vi "Configure Multi DMM.vi"(8 "error in (no error)":errorcluster, 11 "BMC in":refnum<class "BMC.lvclass">) -> (0 "error out":errorcluster, 3 "BMC out":refnum<class "BMC.lvclass">)   [LabVIEW 2012, in "BMC.lvclass"]
uses:
  BMC.lvclass
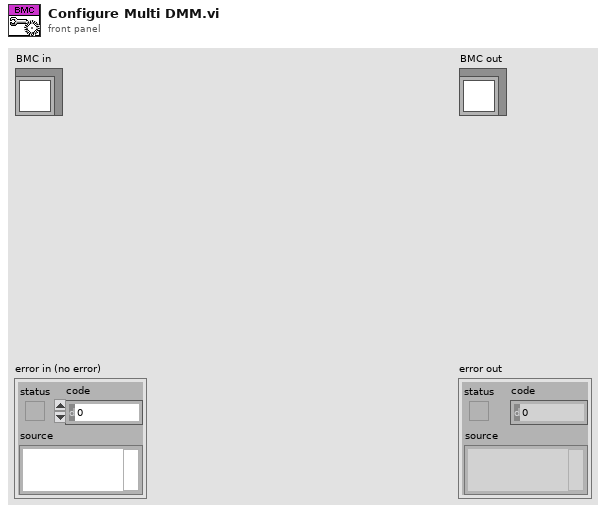
[diagram p1: front panel]
types:
  T1 = enum16{"CIUsb_CONTROL_ASSERT_FRAME_SYNC", "CIUsb_CONTROL_DEASSERT_FRAME_SYNC", "CIUsb_CONTROL_ASSERT_FRESET", "CIUsb_CONTROL_DEASSERT_FRESET", "CIUsb_CONTROL_ASSERT_HV_ENAB", "CIUsb_CONTROL_DEASSERT_HV_ENAB", "CIUsb_CONTROL_ASSERT_LV_SHDN", "CIUsb_CONTROL_DEASSERT_LV_SHDN", "CIUsb_CONTROL_ASSERT_EXT_I2C", "CIUsb_CONTROL_DEASSERT_EXT_I2C", "CIUsb_CONTROL_MINI_MODE"}
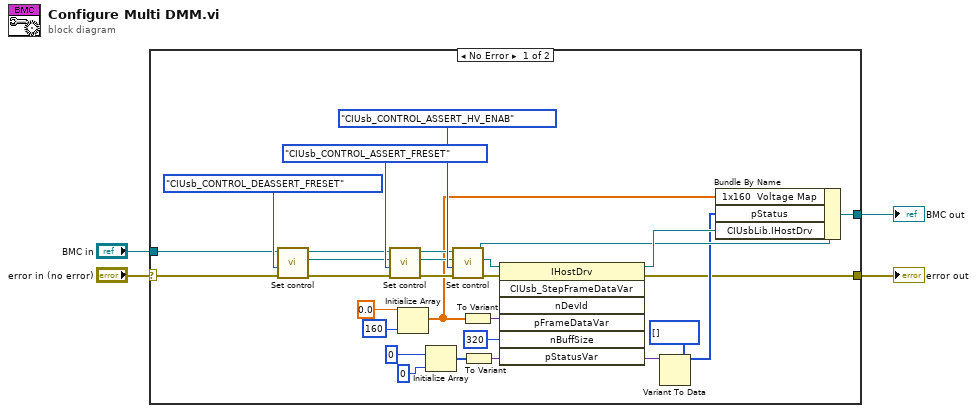
[diagram p0: block diagram]
diagram:
  n1 = case shown="No Error" "error in (no error)" {
    selector: "error in (no error)" -> [w13 w35]
    tunnel: [w12 w35] -> w3
    tunnel: [w10 w34] -> w1
    tunnel: "BMC in" -> [w11 w34]
    frame No Error {
      n2 = call-dynamic "Set control.vi"("BMC in"=w11, "CIUSBLib_SetControl"=T1."CIUsb_CONTROL_DEASSERT_FRESET", "error in (no error)"=w13) -> ("BMC out"=w22:refnum<class "BMC.lvclass">, "CiUsbLib.IHostDrv"=w15:refnum<k7>, "error out"=w26:errorcluster)  [unwired: 5 in]
      n3 = call-dynamic "Set control.vi"("BMC in"=w22, "CIUsbLib.IHostDrv"=w15, "CIUSBLib_SetControl"=T1."CIUsb_CONTROL_ASSERT_FRESET", "error in (no error)"=w26) -> ("BMC out"=w21:refnum<class "BMC.lvclass">, "CiUsbLib.IHostDrv"=w14:refnum<k7>, "error out"=w25:errorcluster)  [unwired: 4 in]
      n4 = Initialize Array(0.0 ("element"), 160 ("dimension size")) -> (w5:dbl[])
      n5 = Initialize Array(0 ("element"), 0 ("dimension size")) -> (w7:i32[])
      n6 = call-dynamic "Set control.vi"("BMC in"=w21, "CIUsbLib.IHostDrv"=w14, "CIUSBLib_SetControl"=T1."CIUsb_CONTROL_ASSERT_HV_ENAB", "error in (no error)"=w25) -> ("BMC out"=w19:refnum<class "BMC.lvclass">, "CiUsbLib.IHostDrv"=w16:refnum<k7>, "error out"=w27:errorcluster)  [unwired: 4 in]
      n7 = To Variant(anything=w5) -> (Variant=w32:variant)
      n8 = To Variant(anything=w7) -> (Variant=w6:variant)
      n9 = invoke class="IHostDrv" method="CIUsb_StepFrameDataVar"(reference=w16, error in=w27, "pFrameDataVar"=w32, "nBuffSize"=320, "pStatusVar"=w6) -> (reference out=w20:refnum<k7>, error out=w12:errorcluster, "pStatusVar"=w29:variant)  [unwired: 2 in, 4 out]
      n10 = Variant To Data(type=i32[] [] ("pStatus"), Variant=w29) -> (data=w17:i32[])  [unwired: 1 in, 1 out]
      n11 = Bundle By Name(cluster=w19, "1x160  Voltage Map"=w5, "pStatus"=w17, "CIUsbLib.IHostDrv"=w20) -> (w10:refnum<class "BMC.lvclass">)
    }
    frame Error {
    }
  }
  "error out" <- w3
  "BMC out" <- w1
